vi "data input.vi"(0 "connection ID":refnum<k5>, 1 "DATA PATTERN":u8, 3 "error in (no error)":errorcluster) -> (6 "connection ID out":refnum<k5>, 7 "output array":u8[](array[numeric]), 8 "New elements/sub array":u32, 9 "error out":errorcluster)   [LabVIEW 2015]
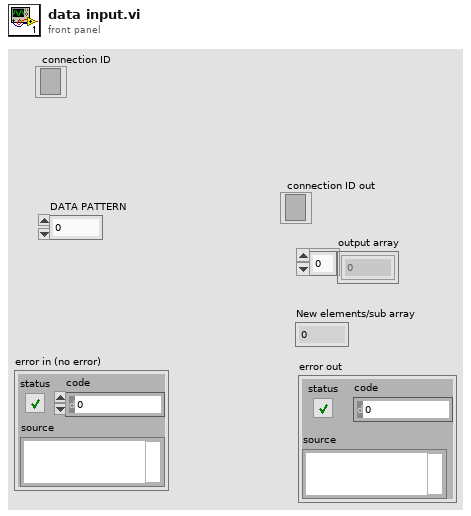
[diagram p1: front panel]
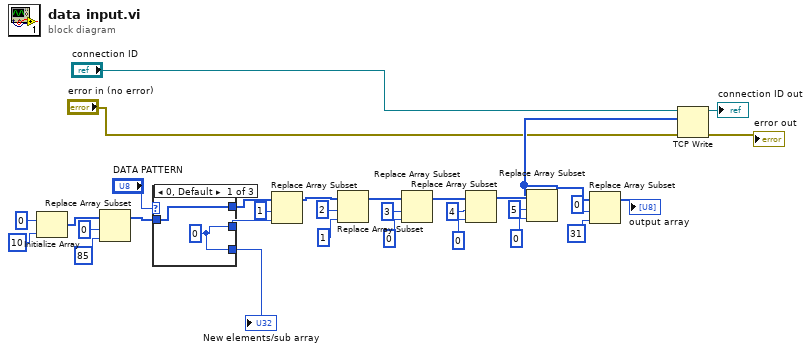
[diagram p0: block diagram]
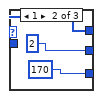
[diagram p2: hidden frame]
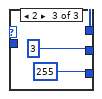
[diagram p3: hidden frame]
diagram:
  n1 = Initialize Array(u8 0 ("元素"), 10 ("维数大小")) -> (w29:u8[])
  n2 = Replace Array Subset(array=w29, new element=u8 85 ("新元素/子数组"), index=0 ("索引")) -> (w26:u8[])
  n3 = case shown="0, Default" "DATA PATTERN" {
    tunnel: w26 -> [w33 w36 w39]
    tunnel: [w33 w36 w39] -> w13
    tunnel: [w32 u8 2 ("新元素/子数组") u8 3 ("新元素/子数组")] -> w7
    tunnel: [w32 u32 170 ("新元素/子数组") u32 255 ("新元素/子数组")] -> w6
    frame 0, Default {
      w32 = u8 0 ("新元素/子数组")
    }
    frame 1 {
    }
    frame 2 {
    }
  }
  "New elements/sub array" <- w6
  n4 = Replace Array Subset(array=w13, new element=w7, index=1 ("索引")) -> (w12:u8[])
  n5 = Replace Array Subset(array=w12, new element=u8 1 ("新元素/子数组"), index=2 ("索引")) -> (w22:u8[])
  n6 = Replace Array Subset(array=w22, new element=u8 0 ("新元素/子数组"), index=3 ("索引")) -> (w19:u8[])
  n7 = Replace Array Subset(array=w19, new element=u8 0 ("新元素/子数组"), index=4 ("索引")) -> (w16:u8[])
  n8 = Replace Array Subset(array=w16, new element=u8 0 ("新元素/子数组"), index=5 ("索引")) -> (w9:u8[])
  n9 = Replace Array Subset(array=w9, new element=u8 31 ("新元素/子数组"), index=0 ("索引")) -> (→"output array":u8[])
  n10 = TCP Write(connection ID="connection ID", data in=w9, error in (no error)="error in (no error)") -> (connection ID out=→"connection ID out":refnum<k5>, error out=→"error out":errorcluster)  [unwired: 1 in, 1 out]
